vi "hydrodynamics method_Old_YCC.vi"() -> ()   [LabVIEW 2014]
uses:
  <vilib>/DAQmx/create/channels.llb/DAQmx Create Channel (AI-Voltage-Basic).vi
  <vilib>/DAQmx/configure/timing.llb/DAQmx Timing (Sample Clock).vi
  <vilib>/DAQmx/read.llb/DAQmx Read (Analog 1D DBL 1Chan NSamp).vi
  <vilib>/Analysis/NI_AALBase.lvlib
  <vilib>/Analysis/3filter.llb/Savitzky-Golay Filter (DBL).vi
  <vilib>/gmath/NI_Gmath.lvlib
  <vilib>/gmath/NumericalOptimization/Nonlinear Curve Fit LM formula string.vi
  Main-Stage-PI/(Global) Current handle and LaserPower_YCC.vi
panel:
  in  "Volumn of glycerol":dbl
  in  "Volumn of water":dbl=1.0
  in  "Temperature (C)":dbl=22.0
  in  "add record time (s)":dbl=0.30000000000000004
  out "best fit parameters":dbl[](array[numeric])
  out "best nonlinear fit (1000X)":dbl[](array[numeric])
  out "QPD (1000X V)":dbl[](array[numeric])
  out "Nor. Counts":dbl[](array[numeric])
  out "dx (nm)":dbl
  out "X Values":dbl[](array[numeric])
  out "Histogram: h(x)":i32[](array[numeric])
  in  "Cut second from initial":dbl=0.2
  in  "side points":i32=6
  out "# of Recorded data point":dbl
  out "Axis":i32
  in  "MultiGaussian Fit?":bool
  in  "Wait between half period (s)":dbl=0.2
  out "Real Current Commanded position (um)":dbl format="%0.5f"
  out "Trap stiffness (pN/nm)":dbl
  out "Drag Force (pN)":dbl
  out "Conversion factor (V/um)":dbl=1.5
  out "dx (V)":dbl
  out "dx2":dbl
  out "dx1":dbl
  in  "bead height (um)":dbl=1.0
  out "Upper QPD":dbl
  out "Lower QPD":dbl
  out "Center QPD":dbl
  out "Time":dbl[](array[numeric])
  in  "Tab Control":T1(tab)
  out "Raw XY Graph":cluster{dbl[], "data":dbl[]}(graph)
  out "Filtered XY Graph":cluster{dbl[], "Filtered X":dbl[]}(graph)
  out "Histogram Graph":T2(graph)
  out "XY Graph":T3(graph)
  in  "Sampling rate (Hz)":dbl=32000.0 format="%0.2f"
  out "traveling time (s)":dbl
  out "True rate?":bool
  in  "T=X\nF=Y":bool
  in  "T= + first\nF=- first":bool
  in  "range  (um)":dbl=20.0 min=0.0 max=100.0 step=0.5 format="%.3f"
  in  "scan rate  (um/s)":dbl=200.0 format="%.3f"
  in  "# of period generate\n(0.5,1,1.5,2...)":dbl
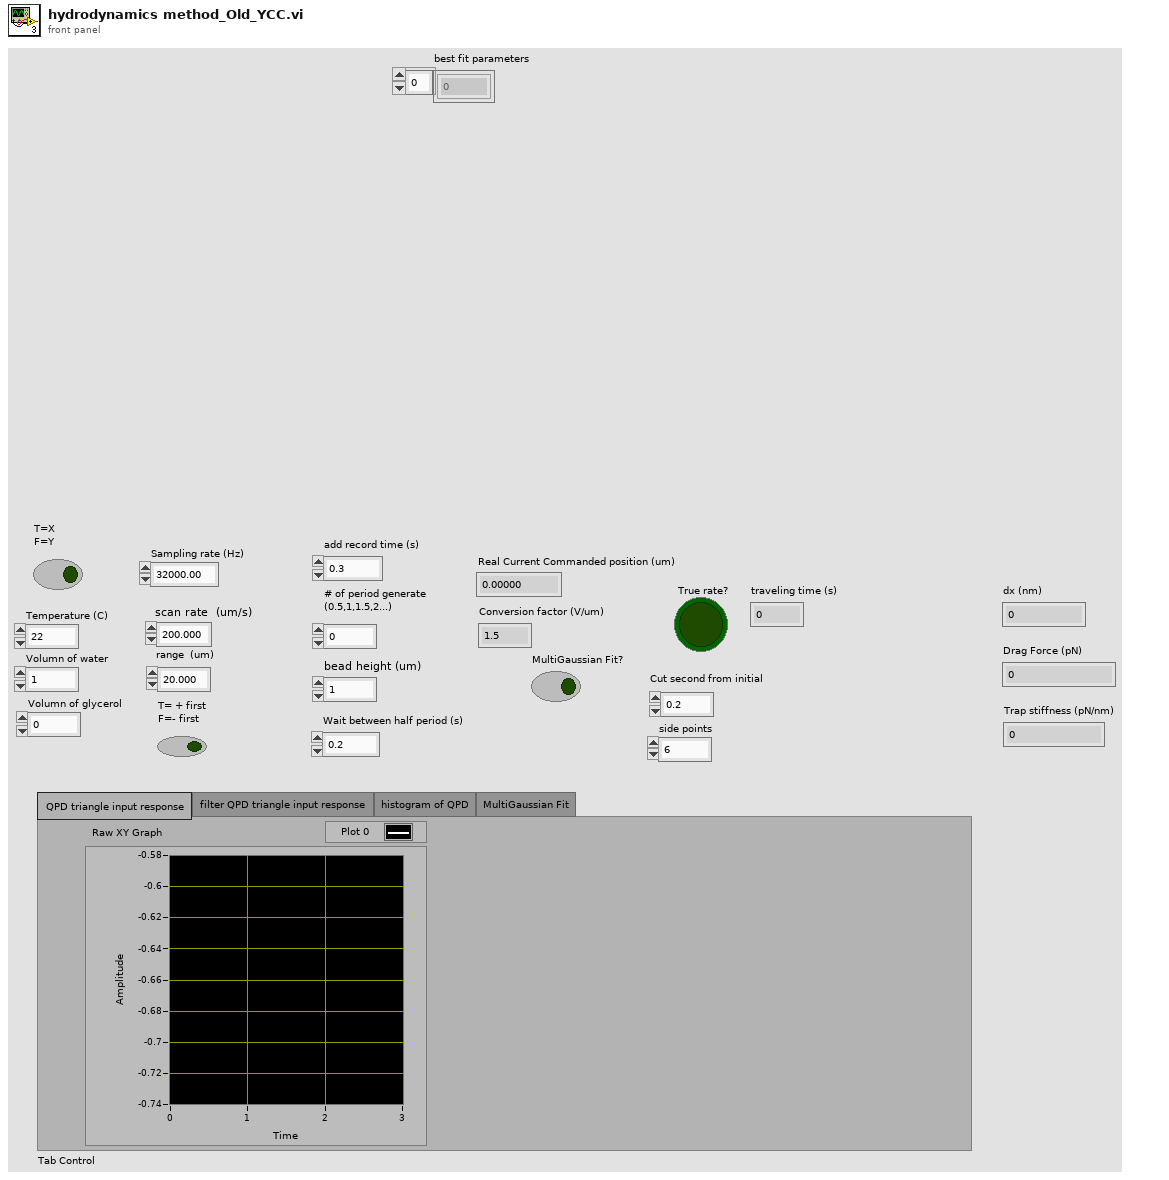
[diagram p1: front panel]
types:
  T1 = enum32{"QPD triangle input response ", "filter QPD triangle input response ", "histogram of QPD", "MultiGaussian Fit"}
  T2 = cluster{"X Values":dbl[], "Histogram: h(x)":i32[]}
  T3 = cluster{"QPD (1000X V)":dbl[], "Nor. Counts":dbl[]}[]
  T4 = cluster{"model":string, "Parameters":string[], "x":string}
  T5 = cluster{"QPD (1000X V)":dbl[], "best nonlinear fit (1000X)":dbl[]}
  T6 = cluster{"QPD (1000X V)":dbl[], "Nor. Counts":dbl[]}
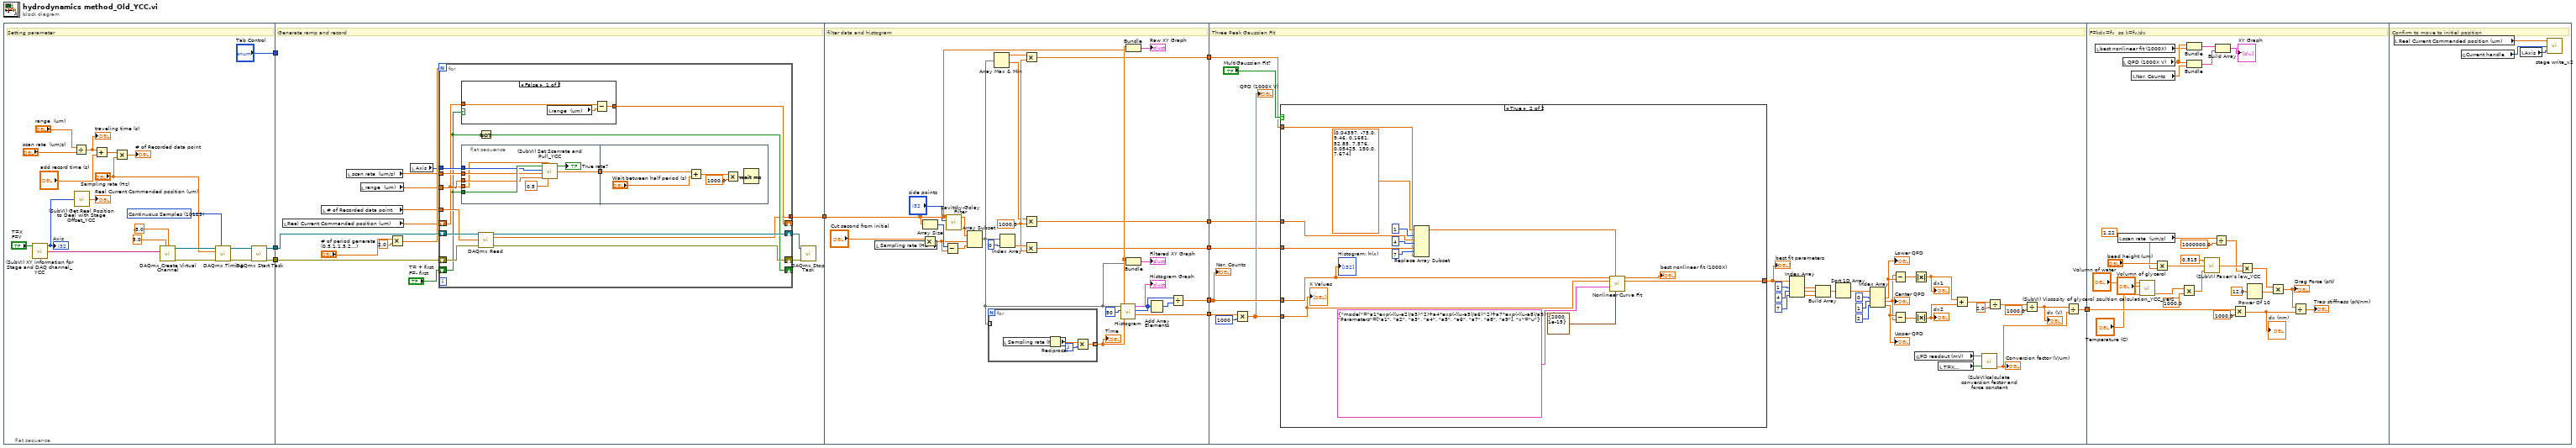
[diagram p0: block diagram]
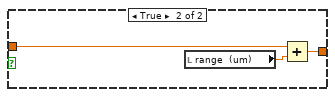
[diagram p2: hidden frame]
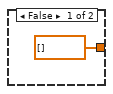
[diagram p3: hidden frame]
diagram:
  n1 = flat-sequence {
    tunnel: [w26] -> w10
    tunnel: [w25] -> w9
    tunnel: ["Tab Control"] -> w8
    tunnel: w10 -> [w45]
    tunnel: w9 -> [w44]
    tunnel: w8 -> [_]
    tunnel: [w43] -> w7
    tunnel: w7 -> [w95]
    tunnel: [w79] -> w6
    tunnel: [w99] -> w5
    tunnel: [w84] -> w3
    tunnel: [w83] -> w2
    tunnel: [w82] -> w1
    tunnel: w6 -> [w144]
    tunnel: w5 -> [w120]
    tunnel: [w122] -> w4
    tunnel: w3 -> [w114]
    tunnel: w2 -> [w113]
    tunnel: w1 -> [w112]
    tunnel: w4 -> [w180]
    frame #0 {
      w31 = 10123 items=["Finite Samples"=10178, "Continuous Samples"=10123, "Hardware Timed Single Point"=12522] ("sample mode")
      # "Setting parameter"
      n2 = call "(SubVI) XY information for Stage and DAQ channel_YCC.vi"("T=X\nF=Y"="T=X\nF=Y") -> ("physical channels"=w23:tag, "Axis"=w13:i32)  [unwired: 3 in]
      "Axis" <- w13
      n3 = Divide(x="range  (um)", y="scan rate  (um/s)") -> (x/y=w18:dbl)
      "traveling time (s)" <- w18
      n4 = call "(SubVI) Get Real Position to Deal with Stage Offset_YCC.vi"("Axis"=w13) -> ("Real Current Commanded position (um)"=→"Real Current Commanded position (um)":dbl)  [unwired: 3 in, 1 out]
      n5 = Add(x=w18, y="add record time (s)") -> (x+y=w17:dbl)
      n6 = Multiply(x=w17, y="Sampling rate (Hz)") -> (x*y=→"# of Recorded data point":dbl)
      n7 = call-poly <vilib>:"DAQmx Create Virtual Channel.vi"("maximum value"=5.0, "minimum value"=-5.0, "physical channels"=w23) -> ("task out"=w29:refnum<k21>, "error out"=w30:errorcluster)  [unwired: 6 in, 5 out]
      n8 = call-poly <vilib>:"DAQmx Timing.vi"("task/channels in"=w29, "sample mode"=w31, "rate"="Sampling rate (Hz)", "error in"=w30) -> ("task out"=w28:refnum<k21>, "error out"=w27:errorcluster)  [unwired: 3 in, 7 out]
      n9 = call <vilib>:"DAQmx Start Task.vi"("task/channels in"=w28, "error in"=w27) -> ("task out"=w26:refnum<k21>, "error out"=w25:errorcluster)  [unwired: 12 out]
    }
    frame #1 {
      # "Generate ramp and record"
      n10 = local read "Real Current Commanded position (um)"() -> (w38:dbl)
      n11 = local read "# of Recorded data point"() -> (w32:dbl)
      n12 = local read "scan rate  (um/s)"() -> (w34:dbl)
      n13 = local read "range  (um)"() -> (w35:dbl)
      n14 = Multiply(x="# of period generate\n(0.5,1,1.5,2...)", y=2.0) -> (x*y=w39:dbl)
      n15 = local read "Axis"() -> (w37:i32)
      n16 = for {
        N: w39 -> [_]
        shift-right: [w57] -> w42
        shift-left: w45 -> [w59]
        shift-right: [w56] -> w41
        shift-left: w44 -> [w58]
        shift-right: [w55] -> _
        shift-left: "T= + first\nF=- first" -> [w48]
        tunnel: w37 -> [w54]
        tunnel: w34 -> [w52]
        tunnel: w35 -> [w51]
        tunnel: w32 -> [w50]
        tunnel: [w49] -> w43 mode=concatenating
        shift-right: [w46] -> _
        shift-left: w38 -> [w47]
        n17 = case shown="False" w48 {
          tunnel: w47 -> [w62 w65]
          tunnel: [w60 w63] -> w46
          frame False {
            n18 = local read "range  (um)"() -> (w61:dbl)
            n19 = Subtract(x=w62, y=w61) -> (x-y=w60:dbl)
          }
          frame True {
            n20 = local read "range  (um)"() -> (w64:dbl)
            n21 = Add(x=w65, y=w64) -> (x+y=w63:dbl)
          }
        }
        n22 = flat-sequence {
          tunnel: w48 -> [w73]
          tunnel: w54 -> [w72]
          tunnel: [w69] -> w53
          tunnel: w52 -> [w68]
          tunnel: w51 -> [w67]
          tunnel: w47 -> [w66]
          tunnel: w53 -> [w78]
          frame #0 {
            n23 = call "(SubVI) Set Scanrate and Pull_YCC.vi"("toward+ ?\nT=+, F=-"=w73, "Start From  (um)"=w66, "axis"=w72, "scan rate  (um/s)"=w68, "waiting time per point (ms)\nrange from 5ms to 0.167 ms"=0.5 ("waiting time per point (ms)\nrange from 5ms to 0.167 ms"), "range  (um)"=w67) -> ("True rate?"=→"True rate?":bool, "traveling time (s)"=w69:dbl)  [unwired: 1 out]
          }
          frame #1 {
            n24 = Add(x=w78, y="Wait between half period (s)") -> (x+y=w77:dbl)
            n25 = Multiply(x=w77, y=1000.0) -> (x*y=w75:dbl)
            n26 = Wait (ms)(milliseconds to wait=w75) -> ()  [unwired: 1 out]
          }
        }
        n27 = Not(x=w48) -> (.not. x?=w55:bool)
        n28 = call-poly <vilib>:"DAQmx Read.vi"("task/channels in"=w59, "number of samples per channel"=w50, "error in"=w58) -> ("task out"=w57:refnum<k21>, "data"=w49:dbl[], "error out"=w56:errorcluster)  [unwired: 1 in, 9 out]
      }
      n29 = call <vilib>:"DAQmx Stop Task.vi"("task/channels in"=w42, "error in"=w41) -> ()  [unwired: 12 in, 2 out]
    }
    frame #2 {
      w87 = 1000.0 ("y")
      # "filter data and histogram"
      n30 = local read "Sampling rate (Hz)"() -> (w96:dbl)
      n31 = Multiply(x="Cut second from initial", y=w96) -> (x*y=w93:dbl)
      n32 = Array Size(array=w95) -> (size(s)=w94:i32)
      n33 = Subtract(x=w94, y=w93) -> (x-y=w92:dbl)
      n34 = call-poly <vilib>:"Savitzky-Golay Filter.vi"("side points"="side points", "X"=w95) -> ("Filtered X"=w91:dbl[])  [unwired: 8 in, 1 out]
      n35 = Array Subset(array=w91, index=w93, length=w92) -> (w89:dbl[])
      n36 = for {
        tunnel: [w105] -> w103 mode=indexing
        tunnel: w89 -> [_] mode=indexing
        i -> [w108]
        n37 = local read "Sampling rate (Hz)"() -> (w107:dbl)
        n38 = Reciprocal(x=w107) -> (1/x=w106:dbl)
        n39 = Multiply(x=w106, y=w108) -> (x*y=w105:dbl)
      }
      "Time" <- w103
      n40 = Array Max & Min(array=w89) -> (max value=w85:dbl, min value=w86:dbl)  [unwired: 2 out]
      n41 = Index Array(array=w89, index=0) -> (element=w88:dbl)
      n42 = Multiply(x=w85, y=w87) -> (x*y=w82:dbl)
      n43 = Multiply(x=w86, y=w87) -> (x*y=w84:dbl)
      n44 = Multiply(x=w88, y=w87) -> (x*y=w83:dbl)
      n45 = call <vilib>:"Histogram.vi"("intervals"=50, "X"=w89) -> ("X Values"=w99:dbl[], "Histogram: h(x)"=w80:i32[], "Histogram Graph"=→"Histogram Graph":T2)  [unwired: 6 in, 1 out]
      n46 = Bundle(w103, "data"=w95) -> (→"Raw XY Graph":cluster{dbl[], "data":dbl[]})  [unwired: 1 in]
      n47 = Bundle(w103, w89) -> (→"Filtered XY Graph":cluster{dbl[], dbl[]})  [unwired: 1 in]
      n48 = Add Array Elements(numeric array=w80) -> (sum=w81:i32)
      n49 = Divide(x=w80, y=w81) -> (x/y=w79:dbl[])
    }
    frame #3 {
      # "Three Peak Gaussian Fit"
      n50 = Multiply(x=w120, y=1000) -> (x*y=w118:dbl[])
      "QPD (1000X V)" <- w118
      n51 = case shown="True" "MultiGaussian Fit?" {
        tunnel: w144 -> [_ w159]
        tunnel: w118 -> [_ w158]
        tunnel: [dbl[] [] ("best nonlinear fit") w147] -> w143
        tunnel: w114 -> [_ w151]
        tunnel: w113 -> [_ w150]
        tunnel: w112 -> [_ w149]
        frame False {
        }
        frame True {
          n52 = Replace Array Subset(array=dbl[] [0.04397, -75.0, 9.46, 0.1681, 52.85, 7.576, 0.05425, 150.0, 7.674] ("initial parameters"), new element #1=w151, index #1=1 ("index"), new element #2=w150, index #2=4 ("index"), new element #3=w149, index #3=7 ("index")) -> (w148:dbl[])
          n53 = call-poly <vilib>:"Nonlinear Curve Fit.vi"("Y"=w159, "initial parameters"=w148, "X"=w158, "model description"=T4 {"model"="a1*exp(-((u-a2)/a3)^2)+a4*exp(-((u-a5)/a6)^2)+a7*exp(-((u-a8)/a9)^2)", "Parameters"=["a1", "a2", "a3", "a4", "a5", "a6", "a7", "a8", "a9"], "x"="u"}, "termination"=cluster{"max iteration":i32, "tolerance":dbl} {"max iteration"=2000, "tolerance"=1e-15}) -> ("best nonlinear fit"=→"best nonlinear fit (1000X)":dbl[], "best fit parameters"=w147:dbl[])  [unwired: 6 in, 3 out]
          "Histogram: h(x)" <- w159
          "X Values" <- w158
        }
      }
      "best fit parameters" <- w143
      n54 = Index Array(array=w143, index #1=1 ("index"), index #2=4 ("index"), index #3=7 ("index")) -> (element #1=w139:dbl, element #2=w138:dbl, element #3=w137:dbl)
      n55 = Build Array(w139, w138, w137) -> (w136:dbl[])
      n56 = Sort 1D Array(array=w136) -> (sorted array=w135:dbl[])
      n57 = Index Array(array=w135, index #1=0 ("index"), index #2=1 ("index"), index #3=2 ("index")) -> (element #1=w131:dbl, element #2=w129:dbl, element #3=w130:dbl)
      "Center QPD" <- w129
      "Lower QPD" <- w131
      "Upper QPD" <- w130
      n58 = Subtract(x=w129, y=w131) -> (x-y=w128:dbl)
      n59 = Subtract(x=w130, y=w129) -> (x-y=w127:dbl)
      n60 = Absolute Value(x=w128) -> (abs(x)=w126:dbl)
      "dx1" <- w126
      n61 = Absolute Value(x=w127) -> (abs(x)=w125:dbl)
      "dx2" <- w125
      n62 = global read "(Global) Current handle and LaserPower_YCC.vi" "PD readout (mV)"() -> (w110)
      n63 = local read "T=X\nF=Y"() -> (w111:bool)
      n64 = Add(x=w126, y=w125) -> (x+y=w124:dbl)
      n65 = call "(SubVI)calculate conversion factor and force constant.vi"("X=T\nY=F"=w111, "laser power (mW)"=w110) -> ("conversion factor (V/um)"=w109:dbl)  [unwired: 2 in, 1 out]
      "Conversion factor (V/um)" <- w109
      n66 = Divide(x=w124, y=2.0) -> (x/y=w117:dbl)
      n67 = Divide(x=w117, y=1000.0) -> (x/y=w115:dbl)
      "dx (V)" <- w115
      n68 = Divide(x=w115, y=w109) -> (x/y=w122:dbl)
      "Nor. Counts" <- w144
    }
    frame #4 {
      # "F=kdx=fv  so k=fv/dx"
      n69 = local read "best nonlinear fit (1000X)"() -> (w175:dbl[])
      n70 = local read "scan rate  (um/s)"() -> (w171:dbl)
      n71 = local read "QPD (1000X V)"() -> (w177:dbl[])
      n72 = local read "Nor. Counts"() -> (w176:dbl[])
      n73 = call "(SubVI) Viscosity of glycerol soultion calculation_YCC_ver2.vi"("Volumn of water"="Volumn of water", "Volumn of glycerol"="Volumn of glycerol", "Temperature (C)"="Temperature (C)") -> ("Viscosity of mix (Pa*s)"=w165:dbl)  [unwired: 4 in, 1 out]
      n74 = Multiply(x="bead height (um)", y=1.22 ("Focal shift factor")) -> (x*y=w166:dbl)
      n75 = Multiply(x=w165, y=1000.0) -> (x*y=w163:dbl)
      n76 = Bundle("QPD (1000X V)"=w177, "best nonlinear fit (1000X)"=w175) -> (w174:T5)  [unwired: 1 in]
      n77 = Bundle("QPD (1000X V)"=w177, "Nor. Counts"=w176) -> (w173:T6)  [unwired: 1 in]
      n78 = call "(SubVI) Faxen's law_YCC.vi"("viscosity (cP)"=w163, "bead height (um)"=w166, "bead radius (um)"=0.515) -> ("Faxen's law of friction coefficient (N/(m/s))"=w186:dbl)  [unwired: 2 in]
      n79 = Divide(x=w171, y=1000000.0) -> (x/y=w169:dbl)
      n80 = Build Array(w174, w173) -> (→"XY Graph":T3)
      n81 = Multiply(x=w180, y=1000.0) -> (x*y=w178:dbl)
      "dx (nm)" <- w178
      n82 = Multiply(x=w186, y=w169) -> (x*y=w185:dbl)
      n83 = Power Of 10(x=12.0) -> (10^x=w183:dbl)
      n84 = Multiply(x=w185, y=w183) -> (x*y=w181:dbl)
      "Drag Force (pN)" <- w181
      n85 = Divide(x=w181, y=w178) -> (x/y=→"Trap stiffness (pN/nm)":dbl)
    }
    frame #5 {
      # "Confirm to move to initial position"
      n86 = local read "Real Current Commanded position (um)"() -> (w190:dbl)
      n87 = global read "(Global) Current handle and LaserPower_YCC.vi" "Current handle"() -> (w189:i32)
      n88 = local read "Axis"() -> (w188:i32)
      n89 = call "stage write_v2.vi"("axis"=w188, "Incoming Handle"=w189, "position"=w190) -> ()  [unwired: 2 in, 1 out]
    }
  }
